vi "grab image_2.vi"(8 "ErrorIn":errorcluster, 9 "Image number":u32, 10 "BuffNr":i16, 11 "ph":u64) -> (0 "output image":dbl[][](array[numeric]) format="%.2f", 1 "error out":errorcluster, 2 "Buffer_Ready":bool, 3 "hout":u64)   [LabVIEW 2014]
uses:
  <vilib>/Platform/TimedLoop/XDataNode/timing_clust.ctl
  <vilib>/Platform/TimedLoop/XDataNode/nitl_modes.ctl
  <vilib>/Platform/TimedLoop/XDataNode/wakeup.ctl
  <vilib>/platform/TimedLoop/XDataNode/XDataNode.xnode
  <vilib>/Platform/TimedLoop/XDataNode/XDNodeRunTimeDep.lvlib
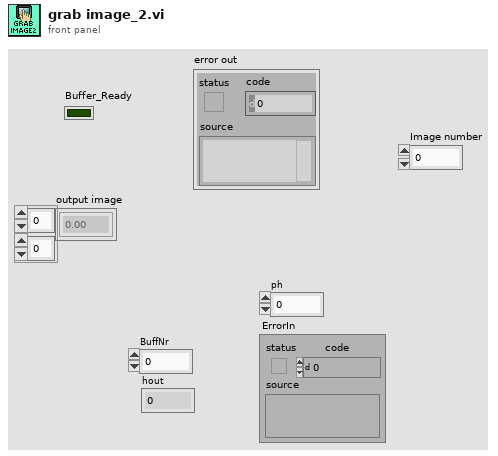
[diagram p1: front panel]
types:
  T1 = typedef "XDNodeRunTimeDep.lvlib/timing_clust.ctl" = cluster{"Expected End [f-1]":u64, "Actual End [f-1]":u64, "Finished Late? [f-1]":bool, "Expected End [i-1]":u64, "Actual End [i-1]":u64, "Finished Late? [i-1]":bool, "Expected Start [i]":u64, "Actual Start [i]":u64, "Expected Start [f]":u64, "Actual Start [f]":u64, "Source Name":string, "Structure Name":string, "Period":i64, "Deadline":i64, "Offset":i64, "Start":i64, "Priority":i32, "Timeout":i32, "Mode":T2, "Wakeup Reason":T3, "Error":errorcluster, "Source Type":string, "Secondary Source Type":string, "Global End Time":u64, "Global Start Time":u64, "Frame Duration":u64, "Iteration Duration":u64, "Assigned CPU":i32, "I/O Scan Engine Mode":u32}
  T2 = typedef "XDNodeRunTimeDep.lvlib/nitl_modes.ctl" = enum32{"No Change", "Process missed periods, maintain original phase", "Discard missed periods, maintain original phase", "Process missed periods, ignore original phase", "Discard missed periods, ignore original phase"}
  T3 = typedef "XDNodeRunTimeDep.lvlib/wakeup.ctl" = enum32{"Normal", "Aborted", "Asynchronous wakeup", "Timing source error", "Timed loop error", "Timeout"}
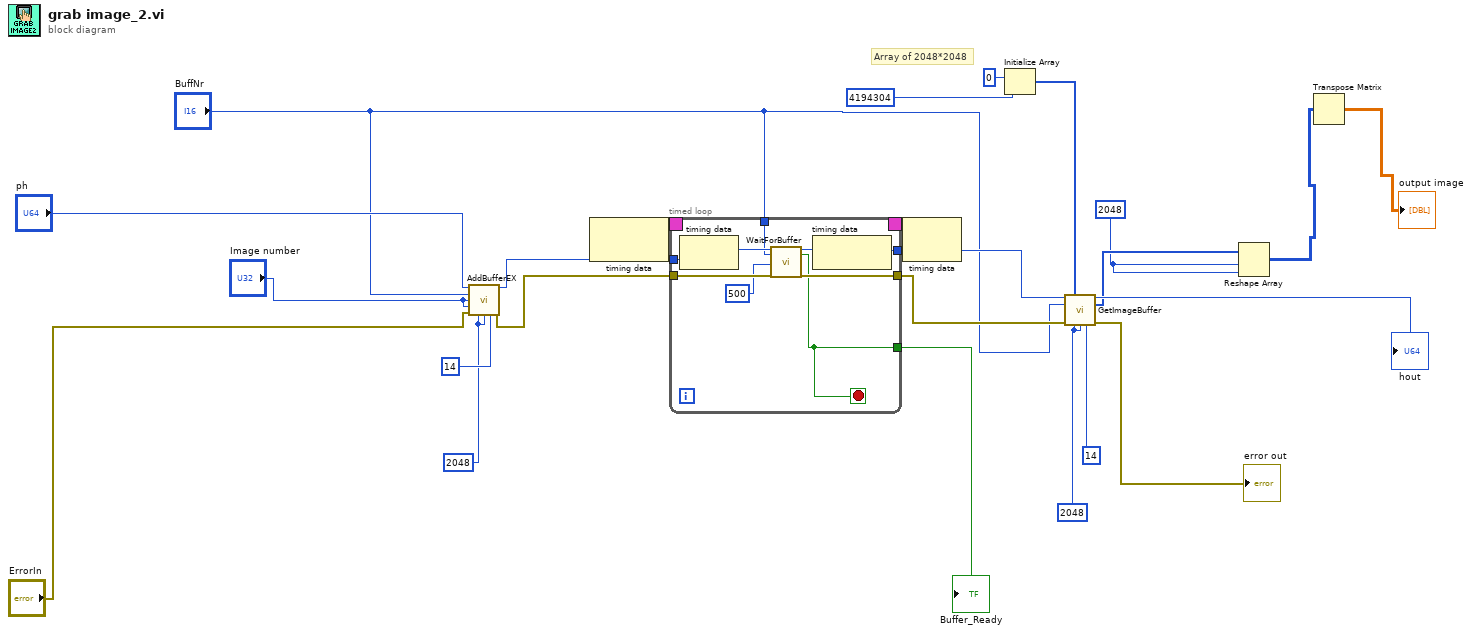
[diagram p0: block diagram]
diagram:
  w6 = u16 2048 ("xRes")
  w14 = 2048
  w18 = u16 2048
  # "Array of 2048*2048"
  n1 = call <userlib>:"AddBufferEX.vi"("ph"="ph", "BuffNr"="BuffNr", "1stImage"="Image number", "LastImage"="Image number", "error in (no error)"="ErrorIn", "XRes"=w18, "YRes"=w18, "BitPerPixel"=u16 14) -> ("hout"=w13:u64, "error out"=w12:errorcluster)  [unwired: 5 in, 1 out]
  n2 = node-c288() -> (w2:T1)  [unwired: 1 in]
  n3 = timed-loop {
    tunnel: w13 -> [w31]
    tunnel: w12 -> [w30]
    tunnel: [w28] -> w17
    tunnel: [w27] -> w16
    tunnel: "BuffNr" -> [w26]
    tunnel: [w25] -> w9
    timing: w2 -> [_]
    timing-out: [_] -> w1
    stop <- w25 stop-if-true
    n4 = node-c288() -> ()  [unwired: 1 in, 1 out]
    n5 = call <userlib>:"WaitForBuffer.vi"("ph"=w31, "sBufNr"=w26, "timeout"=u32 500, "error in (no error)"=w30) -> ("hout"=w28:u64, "Buffer_Ready"=w25:bool, "error out"=w27:errorcluster)  [unwired: 11 in, 2 out]
    n6 = node-c288() -> ()  [unwired: 1 in, 1 out]
  }
  "Buffer_Ready" <- w9
  n7 = node-c288(w1) -> ()  [unwired: 1 out]
  n8 = Initialize Array(i16 0 ("element"), 4194304 ("dimension size")) -> (w21:i16[])
  n9 = call <userlib>:"GetImageBuffer.vi"("ph"=w17, "BuffIn"=w21, "BuffNr"="BuffNr", "error in (no error)"=w16, "xRes"=w6, "yRes"=w6, "Bitresolution"=u16 14 ("BitPerPixel")) -> ("hout"=→"hout":u64, "BuffOut"=w15:u16[], "error out"=→"error out":errorcluster)  [unwired: 5 in, 1 out]
  n10 = Reshape Array(w15, w14, w14) -> (w4:u16[][])
  n11 = Transpose Matrix(1:w4) -> (0:→"output image":dbl[][])
